vi "IMU 3D Display.vi"(8 "Yaw":dbl(knob) scale=0.0..360.0, 9 "Pitch":dbl(knob) scale=0.0..360.0, 10 "Roll":dbl(knob) scale=0.0..360.0, 11 "Color":u32(colorbox)=16711680) -> (3 "3D Picture":refnum<vi>(3d-picture))   [LabVIEW 2014]
uses:
  <vilib>/picture/3D Picture Control/Object/Create Object (name).vi
  <vilib>/picture/3D Picture Control/NI_3D Picture Control.lvlib
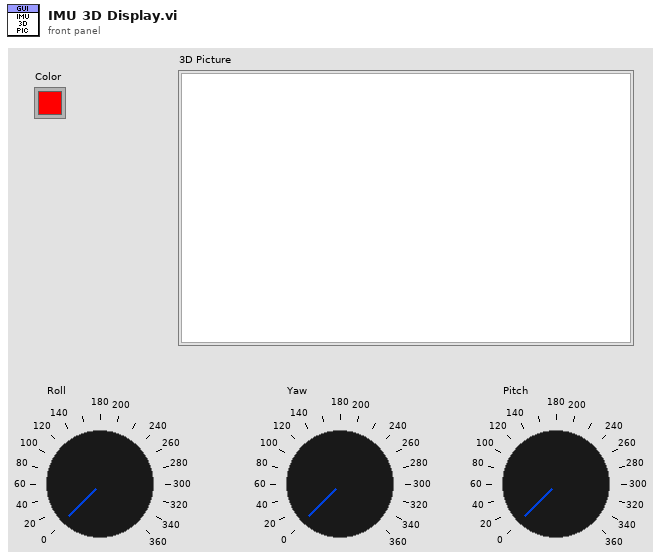
[diagram p1: front panel]
types:
  T1 = cluster{"Red":sgl, "Green":sgl, "Blue":sgl, "Alpha":sgl}
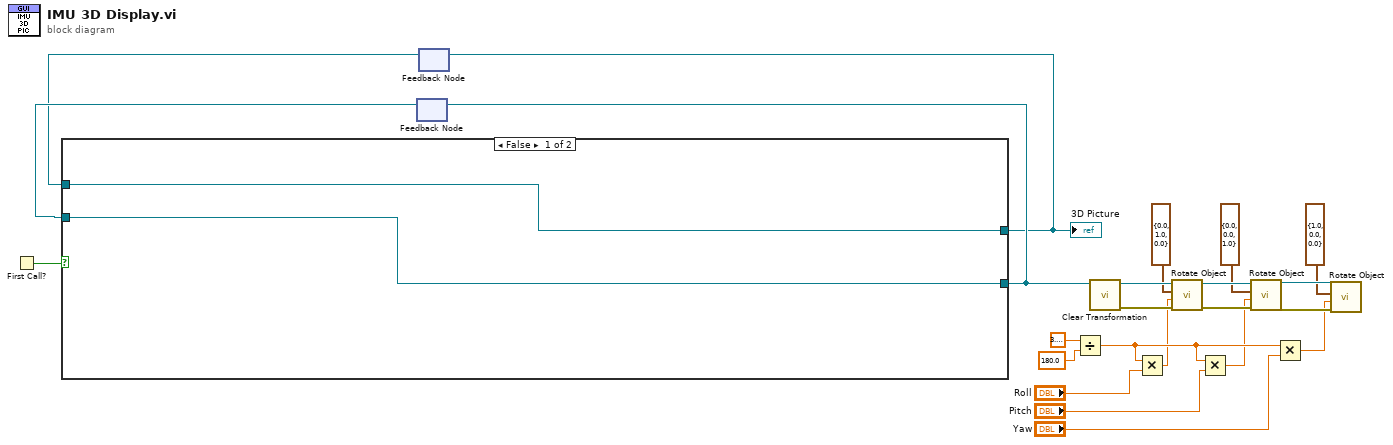
[diagram p0: block diagram]
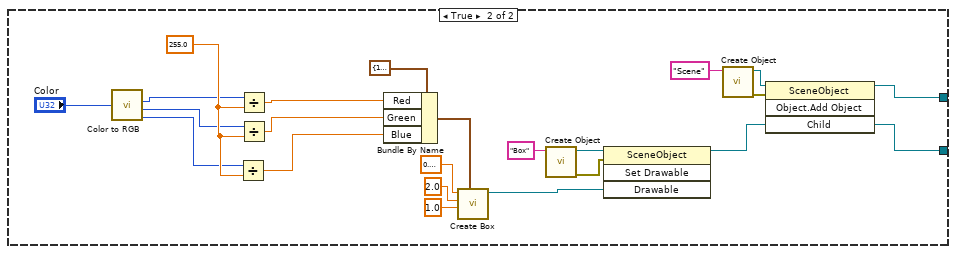
[diagram p2: hidden frame]
diagram:
  n1 = First Call?() -> (First Call?: T/F=w5:bool)
  n2 = feedback #1() -> (w4:refnum<vi>)  [unwired: 1 in]
  n3 = feedback #2() -> (w1:refnum<vi>)  [unwired: 1 in]
  n4 = case shown="False" w5 {
    tunnel: [w25 w27] -> w3
    tunnel: w4 -> [w25 _]
    tunnel: [w24 w26] -> w2
    tunnel: w1 -> [w24 _]
    frame False {
    }
    frame True {
      w38 = 255.0 ("y")
      n5 = call <vilib>:"Color to RGB.vi"("Color"="Color") -> ("R"=w37:u8, "G"=w36:u8, "B"=w35:u8)  [unwired: 1 out]
      n6 = Divide(x=w35, y=w38) -> (x/y=w32:dbl)
      n7 = Divide(x=w37, y=w38) -> (x/y=w34:dbl)
      n8 = Divide(x=w36, y=w38) -> (x/y=w33:dbl)
      n9 = Bundle By Name(cluster=T1 {"Red"=1.0, "Green"=0.0, "Blue"=0.0, "Alpha"=1.0} ("Color"), "Red"=w34, "Green"=w33, "Blue"=w32) -> (w39:T1)
      n10 = call <vilib>:"Create Box.vi"("Color"=w39, "Length Z"=sgl 1.0, "Length Y"=sgl 2.0, "Length X"=sgl 0.2) -> ("New Box Refnum"=w48:refnum<vi>)  [unwired: 6 in, 1 out]
      n11 = call-poly <vilib>:"Create Object.vi"("Name"="Box") -> ("error out"=w47:errorcluster, "Scene:New Object"=w46:refnum<vi>)  [unwired: 9 in]
      n12 = invoke class="SceneObject" method="Set Drawable"(reference=w46, error in=w47, "Drawable"=w48) -> (reference out=w28:refnum<vi>)  [unwired: 1 in, 3 out]
      n13 = call-poly <vilib>:"Create Object.vi"("Name"="Scene") -> ("error out"=w31:errorcluster, "Scene:New Object"=w30:refnum<vi>)  [unwired: 9 in]
      n14 = invoke class="SceneObject" method="Object.Add Object"(reference=w30, error in=w31, "Child"=w28) -> (reference out=w26:refnum<vi>, "Child"=w27:refnum<vi>)  [unwired: 1 in, 2 out]
    }
  }
  "3D Picture" <- w2
  n15 = feedback-in #1(w3) -> ()
  n16 = feedback-in #2(w2) -> ()
  n17 = Divide(x=3.141592653589793, y=180.0) -> (x/y=w12:dbl)
  n18 = call <vilib>:"Clear Transformation.vi"("Object Refnum In"=w3) -> ("error out"=w20:errorcluster, "Object Refnum Out"=w21:refnum<vi>)  [unwired: 9 in]
  n19 = Multiply(x=w12, y="Roll") -> (x*y=w10:dbl)
  n20 = call <vilib>:"Rotate Object.vi"("error in (no error)"=w20, "Angle"=w10, "Axis"=cluster{"X":sgl, "Y":sgl, "Z":sgl} {"X"=0.0, "Y"=1.0, "Z"=0.0}, "Scene.Object In"=w21) -> ("error out"=w22:errorcluster, "Scene.Object Out"=w23:refnum<vi>)  [unwired: 6 in]
  n21 = Multiply(x=w12, y="Pitch") -> (x*y=w9:dbl)
  n22 = call <vilib>:"Rotate Object.vi"("error in (no error)"=w22, "Angle"=w9, "Axis"=cluster{"X":sgl, "Y":sgl, "Z":sgl} {"X"=0.0, "Y"=0.0, "Z"=1.0}, "Scene.Object In"=w23) -> ("error out"=w15:errorcluster, "Scene.Object Out"=w16:refnum<vi>)  [unwired: 6 in]
  n23 = Multiply(x=w12, y="Yaw") -> (x*y=w11:dbl)
  n24 = call <vilib>:"Rotate Object.vi"("error in (no error)"=w15, "Angle"=w11, "Axis"=cluster{"X":sgl, "Y":sgl, "Z":sgl} {"X"=1.0, "Y"=0.0, "Z"=0.0}, "Scene.Object In"=w16) -> ()  [unwired: 6 in, 2 out]
